vi "PVCAM_SetupSeq.vi"(0 "hCam":i16, 1 "exp_mode":i16, 5 "exp_total":u16, 7 "rgn_total":i16, 9 "rgn_type":T1={"s1"=0, "s2"=1199, "sbin"=1, "p1"=0, "p2"=1199, "pbin"=1}, 11 "error in (no error)":errorcluster, 12 "exp_time":u32=10) -> (4 "stream_size":u32, 6 "return type":i16, 15 "error out":errorcluster)   [LabVIEW 2021]
uses:
  PVCAM_rgn_type.ctl
  pvcam64.dll
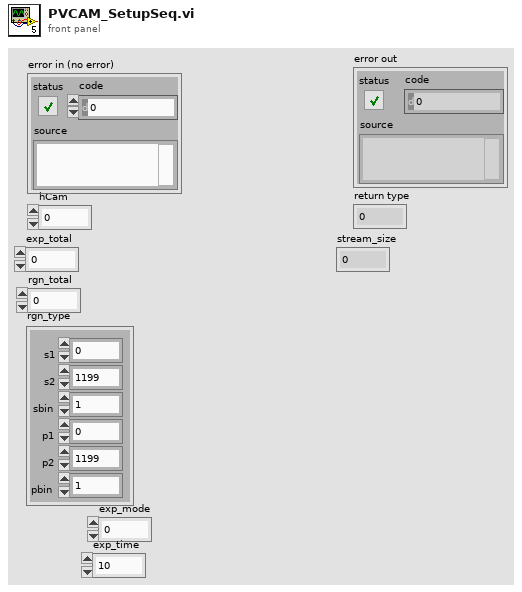
[diagram p1: front panel]
types:
  T1 = typedef "PVCAM_rgn_type.ctl" = cluster{"s1":u16, "s2":u16, "sbin":u16, "p1":u16, "p2":u16, "pbin":u16}
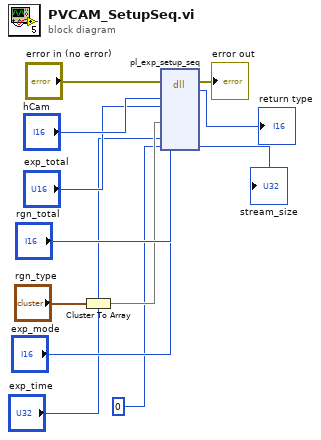
[diagram p0: block diagram]
diagram:
  n1 = Cluster To Array(cluster="rgn_type") -> (array=w5:u16[])
  n2 = dll-call lib="pvcam64.dll" fn="pl_exp_setup_seq"(error in="error in (no error)", "hCam"="hCam", "exp_total"="exp_total", "rgn_total"="rgn_total", "region"=w5, "exp_mode"="exp_mode", "exp_time"="exp_time", "stream_size"=u32 0) -> (error out=→"error out":errorcluster, "return type"=→"return type":i16, "stream_size"=→"stream_size":u32)  [unwired: 8 in, 1 out]
